vi "Shutdown.vi"(8 "error in (no error)":errorcluster, 11 "Nominal Streaming in":refnum<class "Nominal Streaming.lvclass">) -> (0 "error out":errorcluster, 3 "Nominal Streaming out":refnum<class "Nominal Streaming.lvclass">)   [LabVIEW 2020, in "Nominal Streaming.lvclass"]
uses:
  Nominal Streaming.lvclass
  Nominal Streaming.lvclass/Nominal Streaming.ctl
  target/i686-pc-windows-msvc/release/nominal_labview_ffi.dll
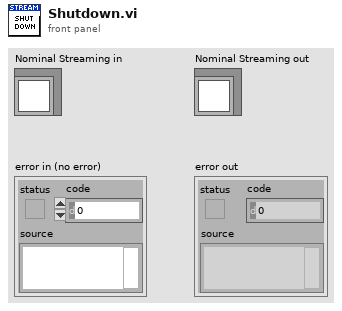
[diagram p1: front panel]
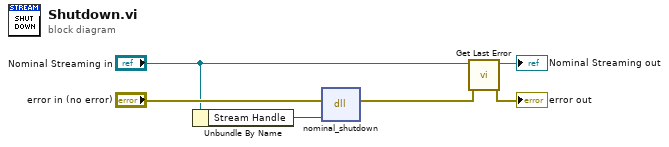
[diagram p0: block diagram]
diagram:
  n1 = Unbundle By Name("Nominal Streaming in") -> ("Stream Handle"=w6:u64)
  n2 = dll-call lib="C:/code/nominal-streaming-labview-ffi/target/i686-pc-windows-msvc/release/nominal_labview_ffi.dll" fn="nominal_shutdown"(error in="error in (no error)", "stream_handle"=w6) -> (error out=w4:errorcluster)  [unwired: 4 in, 1 out]
  n3 = call "Get Last Error.vi"("error in (no error)"=w4, "Nominal Streaming in"="Nominal Streaming in") -> ("error out"=→"error out":errorcluster, "Nominal Streaming out"=→"Nominal Streaming out":refnum<class "Nominal Streaming.lvclass">)  [unwired: 8 in]
